vi "LV FPGA Serial Write.vi"(0 "Write FIFO":refnum<k21>="LIDARRaphaelWriteFIFO", 5 "Transmit":refnum<k21>="Chassis1/Mod4/DIO11", 7 "baud rate (9600)":u32=9600, 9 "data bits (8)":i32=8 min=5 max=8 step=1, 11 "parity (0:none)":enum16{"None", "Odd", "Even", "Mark", "Space"}(ring), 12 "stop bits (10: 1 bit)":u16(ring)=10 items=["1.0"=10, "1.5"=15, "2.0"=20], 13 "Invert Polarity?":bool) -> ()   [LabVIEW 2010]
uses:
  <vilib>/eio/EIONode/EIONode.xnode
  <vilib>/rvi/eio/nirviEIOImplementation/nirviEIOImplementation.xnode
  <vilib>/rvi/eio/common/nirviEmuClasses.ctl
  <vilib>/rvi/DataTransferAndStorage/Container/XNode/niFpgaContainer.xnode
  <vilib>/rvi/DataTransferAndStorage/Container/Common/niFpgaTransferTypeControl.ctl
  <vilib>/rvi/FIFO/Fifo_Types/niFpgaFifoControlLogicControl.ctl
  <vilib>/rvi/DataTransferAndStorage/Container/Common/niFpgaContainerMethod.ctl
  <vilib>/rvi/DataTransferAndStorage/Container/Common/niFpgaContainerMetaDataKey.ctl
  <vilib>/rvi/DataTransferAndStorage/FIFO/niFpgaPeerToPeerStreamState.ctl
  <vilib>/rvi/eio/common/nirviEmuTemplateMethod_noerrors.vi
  <vilib>/rvi/DataTransferAndStorage/Container/Common/niFpgaContainerExecOnDevCompGetState.vi
  <vilib>/rvi/FIFO/Fifo_Resource/nirvififoEmulationSetSize.vi
  <vilib>/rvi/DataTransferAndStorage/Container/Common/niFpgaContainerGetUniqueNameForEmu.vi
  <vilib>/rvi/interface/RandomDataEmulation/nirviRandomDataFPGAFIFO.vi
  <vilib>/rvi/interface/RandomDataEmulation/niFpgaRandomDataHandleErrors.vi
  <vilib>/rvi/eio/common/nirviEmuReportErrorAndStop.vi
panel:
  out "Read: Transmission Error":bool
  in  "stop":bool
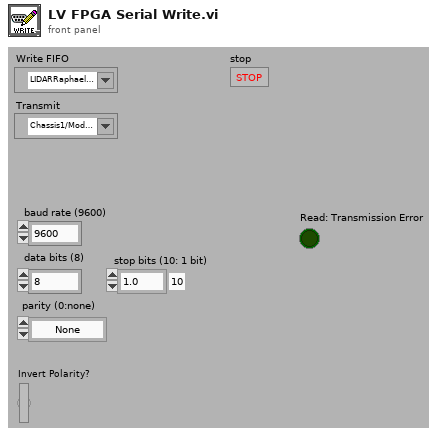
[diagram p1: front panel]
types:
  T1 = typedef "nirviEmuClasses.ctl" = enum16{"IO Read", "IO Write", "Method", "Property Read", "Property Write"}
  T2 = typedef "niFpgaFifoControlLogicControl.ctl" = enum16{"Slice Fabric", "Target Optimal", "Built-in"}
  T3 = typedef "niFpgaContainerMethod.ctl" = enum16{"<none>", "write", "read", "clear", "getNumberOfElementsToWrite", "getNumberOfElementsToRead", "enable", "disable", "flushAndDisable", "getStreamState", "readA", "readB", "dramWrite", "dramWriteWithByteEnables", "dramRequestData", "dramRetrieveData"}
  T4 = typedef "niFpgaTransferTypeControl.ctl" = enum16{"Target-Scoped", "Host to Target - DMA", "Target to Host - DMA", "Peer to Peer Reader", "Peer to Peer Writer", "Bidirectional"}
  T5 = typedef "niFpgaPeerToPeerStreamState.ctl" = enum16{"Unlinked", "Disabled", "Enabled", "Flushing"}
  T6 = typedef "niFpgaContainerMetaDataKey.ctl" = enum16{"FPGA FIFO", "FPGA Memory", "FPGA Register"}
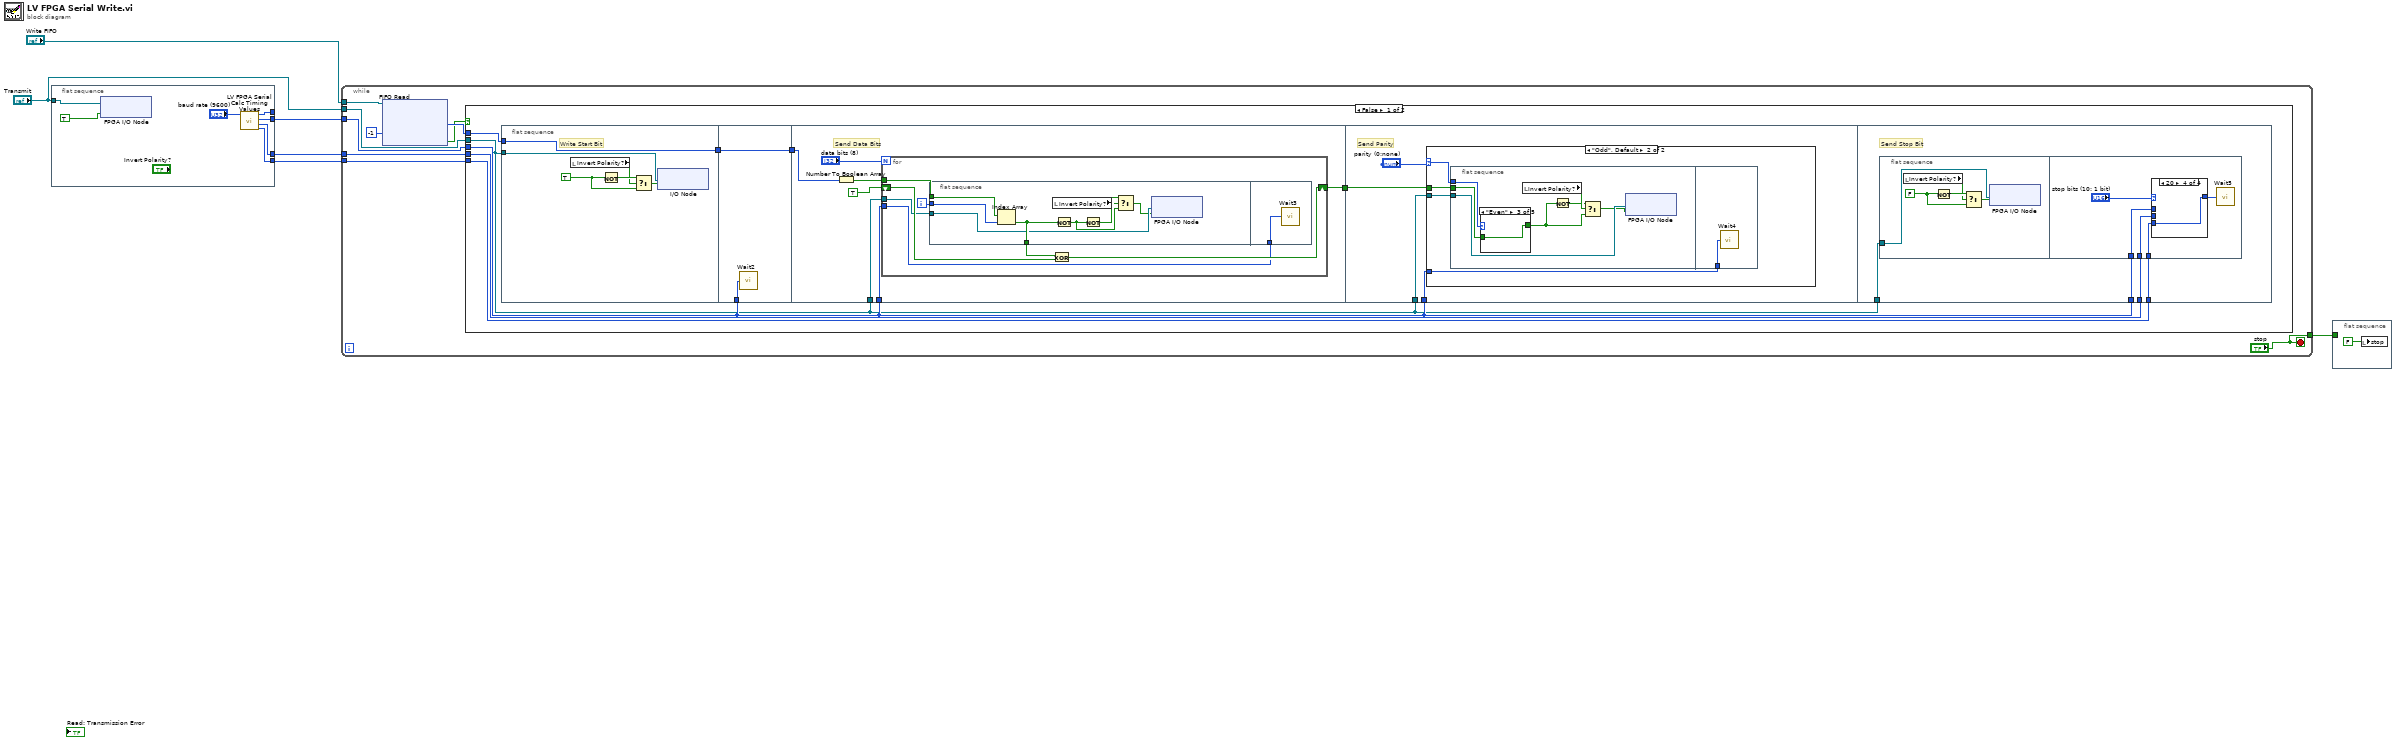
[diagram p0: block diagram]
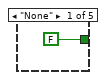
[diagram p3: hidden frame]
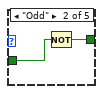
[diagram p4: hidden frame]
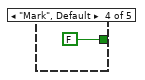
[diagram p5: hidden frame]
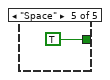
[diagram p6: hidden frame]
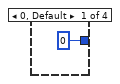
[diagram p7: hidden frame]
diagram:
  n1 = flat-sequence {
    tunnel: [w9] -> w6
    tunnel: [w12] -> _
    tunnel: [w11] -> w5
    tunnel: [w10] -> w4
    tunnel: "Transmit" -> [w7]
    frame #0 {
      n2 = xnode "FPGA I/O Node"("I/O Item"=TRUE ("Digital Enable"), "FPGA I/O In"=w7) -> ()  [unwired: 1 out]
      n3 = call "LV FPGA Serial Calc Timing Values.vi"("baud rate (1000000)"="baud rate (9600)") -> ("Two Bit"=w10:u32, "One and Half Bit"=w11:u32, "One Bit"=w9:u32, "Half Bit"=w12:u32)  [unwired: 1 in, 2 out]
    }
  }
  n4 = while {
    tunnel: w4 -> [w33]
    tunnel: w5 -> [w32]
    tunnel: w6 -> [w31]
    tunnel: "Transmit" -> [w30]
    tunnel: ["stop"] -> w3
    tunnel: "Write FIFO" -> [w25]
    stop <- "stop" stop-if-true
    n5 = xnode ("FIFO Read")("Timeout"=-1, "FIFO In"=w25) -> ("Element"=w29:u8, "Timed Out?"=w27:bool)  [unwired: 1 out]
    n6 = case shown="False" w27 {
      tunnel: w33 -> [w355 _]
      tunnel: w32 -> [w354 _]
      tunnel: w31 -> [w353 _]
      tunnel: w30 -> [w352 _]
      tunnel: w29 -> [w351 _]
      frame False {
        n7 = flat-sequence {
          tunnel: w352 -> [w364]
          tunnel: w351 -> [w359]
          tunnel: [w359] -> w358
          tunnel: w353 -> [w377]
          tunnel: [w376] -> w357
          tunnel: w358 -> [w376]
          tunnel: w353 -> [w384]
          tunnel: [w382] -> w356
          tunnel: w352 -> [w380]
          tunnel: w357 -> [w379]
          tunnel: w353 -> [w414]
          tunnel: w356 -> [w415]
          tunnel: w352 -> [w413]
          tunnel: w353 -> [w448]
          tunnel: w354 -> [w447]
          tunnel: w355 -> [w446]
          tunnel: w352 -> [w445]
          frame #0 {
            w362 = TRUE
            # "Write Start Bit"
            n8 = local read "Invert Polarity?"() -> (w361:bool)
            n9 = Not(x=w362) -> (.not. x?=w363:bool)
            n10 = Select(t=w363, s=w361, f=w362) -> (s? t:f=w360:bool)
            n11 = xnode "I/O Node"("I/O Item"=w360, "FPGA I/O In"=w364) -> ()  [unwired: 1 out]
          }
          frame #1 {
            n12 = call "Wait2"("Count(Ticks)"=w377) -> ()  [unwired: 1 out]
          }
          frame #2 {
            # "Send Data Bits"
            n13 = Number To Boolean Array(number=w379) -> (Boolean array=w381:bool[])
            n14 = for {
              N: "data bits (8)" -> [_]
              tunnel: w384 -> [w388]
              shift-right: [w391] -> w382
              shift-left: TRUE -> [w390]
              tunnel: w381 -> [w387]
              tunnel: w380 -> [w385]
              i -> [w389]
              n15 = flat-sequence {
                tunnel: w389 -> [w399]
                tunnel: w387 -> [w398]
                tunnel: [w397] -> w386
                tunnel: w385 -> [w396]
                tunnel: w388 -> [w411]
                frame #0 {
                  n16 = Index Array(array=w398, index=w399) -> (element=w397:bool)
                  n17 = local read "Invert Polarity?"() -> (w393:bool)
                  n18 = Not(x=w397) -> (.not. x?=w394:bool)
                  n19 = Not(x=w394) -> (.not. x?=w395:bool)
                  n20 = Select(t=w395, s=w393, f=w394) -> (s? t:f=w392:bool)
                  n21 = xnode "FPGA I/O Node"("I/O Item"=w392, "FPGA I/O In"=w396) -> ()  [unwired: 1 out]
                }
                frame #1 {
                  n22 = call "Wait3"("Count(Ticks)"=w411) -> ()  [unwired: 1 out]
                }
              }
              n23 = Exclusive Or(1:w390, 2:w386) -> (0:w391:bool)
            }
          }
          frame #3 {
            # "Send Parity"
            n24 = case shown="\"Odd\", Default" "parity (0:none)" {
              selector: "parity (0:none)" -> [_ w419]
              tunnel: w415 -> [_ w418]
              tunnel: w414 -> [_ w417]
              tunnel: w413 -> [_ w416]
              frame "None" {
              }
              frame "Odd", Default {
                n25 = flat-sequence {
                  tunnel: w418 -> [w425]
                  tunnel: w419 -> [w426]
                  tunnel: w416 -> [w424]
                  tunnel: w417 -> [w444]
                  frame #0 {
                    n26 = case shown="\"Even\"" w426 {
                      tunnel: w425 -> [_ w440 w441 _ _]
                      tunnel: [FALSE ("y") w439 w441 FALSE ("y") TRUE ("y")] -> w421
                      frame "None" {
                      }
                      frame "Odd" {
                        n27 = Not(x=w440) -> (.not. x?=w439:bool)
                      }
                      frame "Even" {
                      }
                      frame "Mark", Default {
                      }
                      frame "Space" {
                      }
                    }
                    n28 = local read "Invert Polarity?"() -> (w423:bool)
                    n29 = Not(x=w421) -> (.not. x?=w422:bool)
                    n30 = Select(t=w422, s=w423, f=w421) -> (s? t:f=w420:bool)
                    n31 = xnode "FPGA I/O Node"("I/O Item"=w420, "FPGA I/O In"=w424) -> ()  [unwired: 1 out]
                  }
                  frame #1 {
                    n32 = call "Wait4"("Count(Ticks)"=w444) -> ()  [unwired: 1 out]
                  }
                }
              }
            }
          }
          frame #4 {
            # "Send Stop Bit"
            n33 = flat-sequence {
              tunnel: w445 -> [w453]
              tunnel: w448 -> [w469]
              tunnel: w447 -> [w468]
              tunnel: w446 -> [w467]
              frame #0 {
                w451 = FALSE
                n34 = local read "Invert Polarity?"() -> (w450:bool)
                n35 = Not(x=w451) -> (.not. x?=w452:bool)
                n36 = Select(t=w452, s=w450, f=w451) -> (s? t:f=w449:bool)
                n37 = xnode "FPGA I/O Node"("I/O Item"=w449, "FPGA I/O In"=w453) -> ()  [unwired: 1 out]
              }
              frame #1 {
                n38 = case shown="20" "stop bits (10: 1 bit)" {
                  tunnel: w469 -> [_ w471 _ _]
                  tunnel: w468 -> [_ _ w472 _]
                  tunnel: w467 -> [_ _ _ w473]
                  tunnel: [u32 0 ("One Bit") w471 w472 w473] -> w466
                  frame 0, Default {
                  }
                  frame 10 {
                  }
                  frame 15 {
                  }
                  frame 20 {
                  }
                }
                n39 = call "Wait5"("Count(Ticks)"=w466) -> ()  [unwired: 1 out]
              }
            }
          }
        }
      }
      frame True {
      }
    }
  }
  n40 = flat-sequence {
    tunnel: w3 -> [_]
    frame #0 {
      n41 = local write "stop"(FALSE ("stop")) -> ()
    }
  }
